vi "svfa_Process Cross Power Subset.vi"(0 "Windowed signal [X]":waveform(dbl)={"t0"=timestamp(0 s since 1904-01-01), "dt"=1.953125e-05, "Y"=[]}, 1 "Windowed signal [Y]":waveform(dbl)={"t0"=timestamp(0 s since 1904-01-01), "dt"=1.953125e-05, "Y"=[]}, 2 "window":u16(ring)=1 items=["None "=0, "Hanning"=1, "Hamming"=2, "Blackman-Harris"=3, "Exact Blackman"=4, "Blackman"=5, "Flat Top"=6, "4 Term B-Harris "=7, "7 Term B-Harris"=8, "Low Sidelobe"=9, "Force - Exponential"=10, "Gaussian"=62], 3 "force/exp settings":T8={"force window [%]"=50.0, "exponential window [%]"=10.0} {"exponential window [%]" min=0.0 max=100.0 format="%.2f"; "force window [%]" min=0.0 max=100.0 format="%.2f"}, 4 "averaging parameters":T11={"averaging mode"=enum."No averaging", "weighting mode"=enum."Linear", "number of averages"=10, "linear mode"=enum."Auto restart"}, 5 "error in (no error)":errorcluster, 6 "Spectrum Settings":T9 {"stop frequency" format="%.2f"; "start frequency" format="%.2f"}, 7 "processing control":T7(ring), 9 "spectrum info in":T1={"channel name"="", "description"="", "x-axis units"=0, "spectral info"={"spectrum type"=enum."Power [Magnitude^2]", "linear/dB"=enum."linear", "window"=0, "window size"=0, "FFT size"=0}, "engineering units"=0, "custom label"="", "dB reference [EU]"=0.0, "peak units"=enum."rms", "weighting filter"=0, "spectral density?"=FALSE, "unit label"="", "spectrum skewed?"=FALSE, "complimentary spectrum units"=enum."none"} {"x-axis units" items=["Time (s)"=0, "Frequency-CB (Hz)"=1, "Frequency-CPB (Hz)"=1248, "Frequency-Arbitrary (Hz)"=2357, "Quefrency (s)"=2, "Revolutions (rev)"=3, "Order"=4, "Speed (RPM)"=11, "Speed (rad/s)"=21, "Index"=65535]; "weighting filter" items=["Linear", "A-weighting", "B-weighting", "C-weighting", "ITU-R 468-4", "Dolby", "CCITT", "C-message", "Wb", "Wc", "Wd", "We", "Wf", "Wh", "Wj", "Wk", "Wm", "AES17 20 kHz lowpass", "AES17 40 kHz lowpass", "AES17 20 kHz highpass", "AES17 40 kHz highpass"]; "dB reference [EU]" format="%.2f"; "engineering units" items=["custom..."=0, "V"=1, "A"=21, "C"=30, "pC"=31, "s"=32, "-"=29, "Pa"=2, "N"=20, "g"=3, "m/s^2"=4, "m/s"=5, "m"=6, "mm/s"=12, "mm"=13, "micron/s"=14, "micron"=15, "in/s^2"=7, "in/s"=8, "in"=9, "mil/s"=10, "mil"=11, "rad/s^2"=16, "rad/s"=17, "rad"=18, "deg/s^2"=26, "deg/s"=27, "deg"=28, "RPM"=22, "cycle/s^2"=23, "Hz"=24, "cycle"=25, "strain"=19]; "spectral info"."window" items=["None "=0, "Hanning"=1, "Hamming"=2, "Blackman-Harris"=3, "Exact Blackman"=4, "Blackman"=5, "Flat Top"=6, "4 Term B-Harris "=7, "7 Term B-Harris"=8, "Low Sidelobe"=9, "Force - Exponential"=10, "Gaussian"=62]}) -> (12 "averages completed":dbl format="%.2f", 13 "processing control":T7(ring), 14 "complex spectrum":T10={"f0"=0.0, "df"=1.0, "complex spectrum"=[]} {"complex spectrum" format="%.2f"; "df" format="%.2f"; "f0" format="%.2f"}, 17 "averaging done":bool, 18 "spectrum info out":T1={"channel name"="", "description"="", "x-axis units"=0, "spectral info"={"spectrum type"=enum."Power [Magnitude^2]", "linear/dB"=enum."linear", "window"=0, "window size"=0, "FFT size"=0}, "engineering units"=0, "custom label"="", "dB reference [EU]"=0.0, "peak units"=enum."rms", "weighting filter"=0, "spectral density?"=FALSE, "unit label"="", "spectrum skewed?"=FALSE, "complimentary spectrum units"=enum."none"} {"x-axis units" items=["Time (s)"=0, "Frequency-CB (Hz)"=1, "Frequency-CPB (Hz)"=1248, "Frequency-Arbitrary (Hz)"=2357, "Quefrency (s)"=2, "Revolutions (rev)"=3, "Order"=4, "Speed (RPM)"=11, "Speed (rad/s)"=21, "Index"=65535]; "weighting filter" items=["Linear", "A-weighting", "B-weighting", "C-weighting", "ITU-R 468-4", "Dolby", "CCITT", "C-message", "Wb", "Wc", "Wd", "We", "Wf", "Wh", "Wj", "Wk", "Wm", "AES17 20 kHz lowpass", "AES17 40 kHz lowpass", "AES17 20 kHz highpass", "AES17 40 kHz highpass"]; "dB reference [EU]" format="%.2f"; "engineering units" items=["custom..."=0, "V"=1, "A"=21, "C"=30, "pC"=31, "s"=32, "-"=29, "Pa"=2, "N"=20, "g"=3, "m/s^2"=4, "m/s"=5, "m"=6, "mm/s"=12, "mm"=13, "micron/s"=14, "micron"=15, "in/s^2"=7, "in/s"=8, "in"=9, "mil/s"=10, "mil"=11, "rad/s^2"=16, "rad/s"=17, "rad"=18, "deg/s^2"=26, "deg/s"=27, "deg"=28, "RPM"=22, "cycle/s^2"=23, "Hz"=24, "cycle"=25, "strain"=19]; "spectral info"."window" items=["None "=0, "Hanning"=1, "Hamming"=2, "Blackman-Harris"=3, "Exact Blackman"=4, "Blackman"=5, "Flat Top"=6, "4 Term B-Harris "=7, "7 Term B-Harris"=8, "Low Sidelobe"=9, "Force - Exponential"=10, "Gaussian"=62]}, 19 "error out":errorcluster)   [LabVIEW 2017]
uses:
  <vilib>/addons/_NISVFA/_Shared subVIs/Controls/svc_Spectrum Info.ctl
  <vilib>/addons/_NISVFA/_Shared subVIs/Controls/svc_X-Axis Units.ctl
  <vilib>/addons/_NISVFA/_Shared subVIs/Controls/svc_Spectrum Type.ctl
  <vilib>/addons/_NISVFA/_Shared subVIs/Controls/svc_Engineering Units Text Ring.ctl
  <vilib>/addons/_NISVFA/_Shared subVIs/Controls/svc_Weighting Filter Text Ring.ctl
  <vilib>/addons/_NISVFA/_Shared subVIs/Controls/svc_Complimentary Spectrum Units.ctl
  <vilib>/addons/_NISVFA/_Shared subVIs/Windowing/svfa_Scaled Time Domain Window (1 Ch).vi
  <vilib>/addons/_NISVFA/_Shared subVIs/Windowing/svfa_Scaled Time Domain Window (Array).vi
  <vilib>/Analysis/4window.llb/Force Window.vi
  <vilib>/Analysis/4window.llb/Force Window (DBL).vi
  <vilib>/Analysis/4window.llb/Exponential Window.vi
  <vilib>/Analysis/4window.llb/Exponential Window (DBL).vi
  <vilib>/Utility/error.llb/Error Cluster From Error Code.vi
  <vilib>/Analysis/0measdsp.llb/Scaled Time Domain Window.vi
  <vilib>/Analysis/0measdsp.llb/Scaled Time Domain Window (DBL).vi
  <vilib>/addons/_NISVFA/_Spectrum Processing/subVIs/svfa_Spectrum Info Window to windowTd Type Def.vi
  <vilib>/addons/_NISVFA/_Shared subVIs/Common/svc_Window Parameters.vi
  <vilib>/addons/_NISVFA/_Shared subVIs/Common/svc_Get Window Info.vi
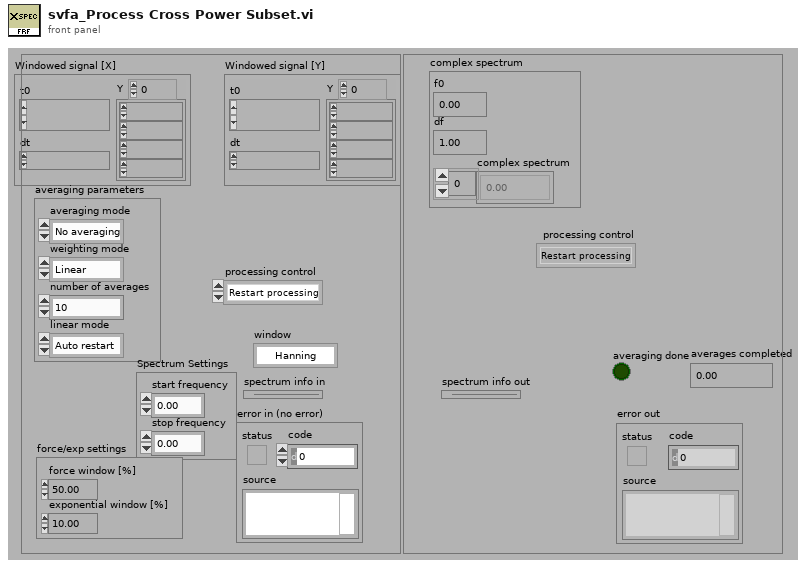
[diagram p1: front panel]
types:
  T1 = typedef "svc_Spectrum Info.ctl" = cluster{"channel name":string, "description":string, "x-axis units":T2, "spectral info":cluster{"spectrum type":T3, "linear/dB":enum16{"linear", "dB"}, "window":u16, "window size":i32, "FFT size":i32}, "engineering units":T4, "custom label":string, "dB reference [EU]":dbl, "peak units":enum16{"rms", "peak", "peak-peak"}, "weighting filter":T5, "spectral density?":bool, "unit label":string, "spectrum skewed?":bool, "complimentary spectrum units":T6}
  T2 = typedef "svc_X-Axis Units.ctl" = u16
  T3 = typedef "svc_Spectrum Type.ctl" = enum16{"FFT Spectrum [complex]", "Amplitude [Magnitude]", "Power [Magnitude^2]", "Cross Spectrum [complex]", "Frequency Response [Complex]"}
  T4 = typedef "svc_Engineering Units Text Ring.ctl" = u16
  T5 = typedef "svc_Weighting Filter Text Ring.ctl" = u16
  T6 = typedef "svc_Complimentary Spectrum Units.ctl" = enum16{"none", "radians", "degrees", "cycles", "imaginary"}
  T7 = enum16{"Restart processing", "Continue processing", "Skip processing"}
  T8 = cluster{"force window [%]":dbl, "exponential window [%]":dbl}
  T9 = cluster{"start frequency":dbl, "stop frequency":dbl}
  T10 = cluster{"f0":dbl, "df":dbl, "complex spectrum":cdb[]}
  T11 = cluster{"averaging mode":enum16{"No averaging", "Vector averaging", "RMS averaging", "Peak hold"}, "weighting mode":enum16{"Linear", "Exponential"}, "number of averages":u32, "linear mode":enum16{"One shot", "Auto restart"}}
  T12 = typedef "svc_Window [Dual FFT].ctl" = u32
  T13 = cluster{"complex spectrum":cluster{"f0":dbl, "df":dbl, "complex spectrum":cdb[]}, "spectrum info":T1}
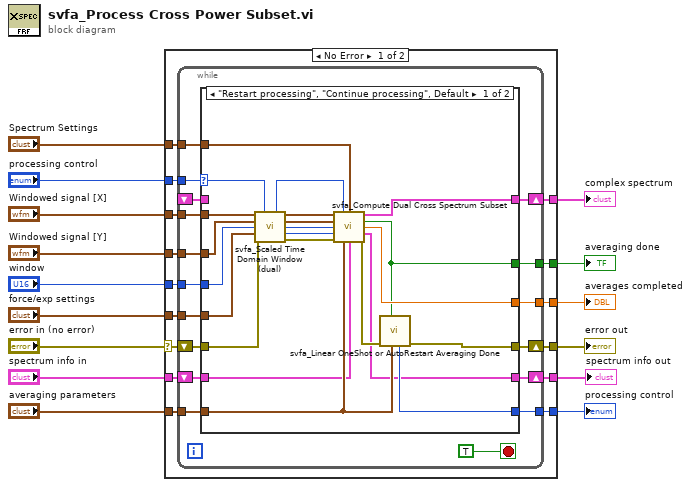
[diagram p0: block diagram]
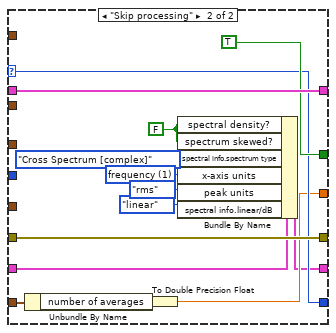
[diagram p2: hidden frame]
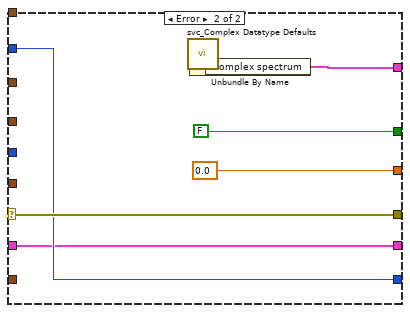
[diagram p3: hidden frame]
diagram:
  n1 = case shown="No Error" "error in (no error)" {
    selector: "error in (no error)" -> [w30 w90]
    tunnel: "averaging parameters" -> [w22 _]
    tunnel: [w29 0.0 ("averages completed")] -> w13
    tunnel: [w24 FALSE ("averaging done")] -> w12
    tunnel: [w18 w85] -> w10
    tunnel: "Windowed signal [X]" -> [w28 _]
    tunnel: "Windowed signal [Y]" -> [w27 _]
    tunnel: "Spectrum Settings" -> [w19 _]
    tunnel: "processing control" -> [w20 w87]
    tunnel: "window" -> [w26 _]
    tunnel: "force/exp settings" -> [w25 _]
    tunnel: [w23 w87] -> w3
    tunnel: "spectrum info in" -> [w17 w84]
    tunnel: [w16 w84] -> w1
    tunnel: [w21 w90] -> w15
    frame No Error {
      n2 = while {
        shift-left: _ -> [w33]
        shift-right: [w34] -> w18
        tunnel: w19 -> [w37]
        tunnel: w20 -> [w36]
        tunnel: w22 -> [w39]
        tunnel: [w40] -> w23
        tunnel: [w41] -> w24
        tunnel: w25 -> [w42]
        tunnel: w26 -> [w43]
        tunnel: w27 -> [w44]
        tunnel: w28 -> [w45]
        tunnel: [w46] -> w29
        shift-right: [w31] -> w16
        shift-left: w17 -> [w32]
        shift-right: [w38] -> w21
        shift-left: w30 -> [w47]
        stop <- TRUE stop-if-true
        n3 = case shown="\"Restart processing\", \"Continue processing\", Default" w36 {
          selector: w36 -> [w52 w80]
          tunnel: [w50 w83] -> w34
          tunnel: w47 -> [w66 w82]
          tunnel: [w65 w77] -> w46
          tunnel: w45 -> [w64 _]
          tunnel: w44 -> [w63 _]
          tunnel: w43 -> [w51 _]
          tunnel: w42 -> [w62 _]
          tunnel: [w61 TRUE ("averaging done")] -> w41
          tunnel: [w60 w80] -> w40
          tunnel: w39 -> [w57 w79]
          tunnel: w37 -> [w54 _]
          tunnel: w33 -> [_ w83]
          tunnel: w32 -> [w49 w71]
          tunnel: [w48 w70] -> w31
          tunnel: [w55 w82] -> w38
          frame "Restart processing", "Continue processing", Default {
            n4 = call <vilib>:"svfa_Scaled Time Domain Window (dual).vi"("Signal in [X]"=w64, "processing control"=w52, "Signal in [Y]"=w63, "window"=w51, "force/exp settings"=w62, "error in (no error)"=w66) -> ("dup processing control"=w53:T7, "Windowed signal [X]"=w69:waveform(dbl), "Windowed signal [Y]"=w68:waveform(dbl), "window"=w59:T12, "window size"=w58:i32, "error out"=w67:errorcluster)  [unwired: 3 in, 1 out]
            n5 = call <vilib>:"svfa_Compute Dual Cross Spectrum Subset.vi"("Windowed signal [X]"=w69, "processing control"=w53, "Spectrum Settings"=w54, "Windowed signal [Y]"=w68, "window"=w59, "window size"=w58, "error in"=w67, "averaging parameters"=w57, "spectrum info in"=w49) -> ("complex spectrum"=w50:T10, "averaging done"=w61:bool, "averages completed"=w65:dbl, "spectrum info out"=w48:T1, "error out"=w56:errorcluster)  [unwired: 2 in]
            n6 = call <vilib>:"svfa_Linear OneShot or AutoRestart Averaging Done.vi"("averaging parameters"=w57, "averaging done"=w61, "error in (no error)"=w56) -> ("error out"=w55:errorcluster, "processing control"=w60:T7)  [unwired: 7 in]
          }
          frame "Skip processing" {
            w72 = u16 1 items=["time"=0, "frequency"=1, "quefrency"=2, "revolutions"=3, "order"=4, "rpm"=11] ("x-axis units")
            w74 = FALSE ("spectral density?")
            n7 = Unbundle By Name(w79) -> ("number of averages"=w78:u32)
            n8 = To Double Precision Float(number=w78) -> (double precision float=w77:dbl)
            n9 = Bundle By Name(cluster=w71, "spectral density?"=w74, "spectrum skewed?"=w74, "spectral info.spectrum type"=svc_Spectrum_Type."Cross Spectrum [complex]", "x-axis units"=w72, "peak units"=enum16{"rms", "peak", "peak-peak"}."rms", "spectral info.linear/dB"=enum16{"linear", "dB"}."linear") -> (w70:T1)
          }
        }
      }
    }
    frame Error {
      n10 = call <vilib>:"svc_Complex Datatype Defaults.vi"() -> ("complex spectrum"=w86:T13)  [unwired: 11 in, 8 out]
      n11 = Unbundle By Name(w86) -> ("complex spectrum"=w85:T10)
    }
  }
  "error out" <- w15
  "averages completed" <- w13
  "averaging done" <- w12
  "complex spectrum" <- w10
  "processing control" <- w3
  "spectrum info out" <- w1
